vi "XaxisFreq.vi"(5 "Start Frequency":dbl, 7 "Stop Frequency":dbl, 9 "Points":dbl) -> (8 "X-Axis":dbl[](array[numeric]))   [LabVIEW 2018]
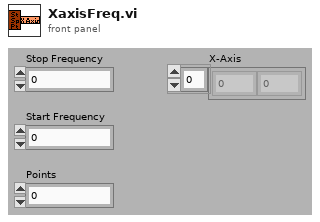
[diagram p1: front panel]
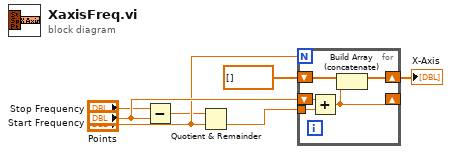
[diagram p0: block diagram]
diagram:
  n1 = Subtract(x="Stop Frequency", y="Start Frequency") -> (x-y=w2:dbl)
  n2 = Quotient & Remainder(x=w2, y="Points") -> (floor(x/y)=w4:dbl)  [unwired: 1 out]
  n3 = for {
    N: "Points" -> [_]
    tunnel: w4 -> [w12]
    shift-right: [w9] -> w7
    shift-left: dbl[] [] -> [w10]
    shift-right: [w8] -> _
    shift-left: "Start Frequency" -> [w11]
    n4 = Add(x=w11, y=w12) -> (x+y=w8:dbl)
    n5 = Build Array (concatenate)(w10, w8) -> (w9:dbl[])
  }
  "X-Axis" <- w7
